vi "Process Libraries.vi"(8 "error in (no error)":errorcluster {"code" format="Error %.0f"}, 10 "Libraries":refnum<class "Library Documentation.lvclass">[](array[class]), 11 "VIDoc Printer In":refnum<class "VIDoc Printer.lvclass">) -> (0 "error out":errorcluster {"code" format="Error %.0f"}, 3 "VIDoc Printer Out":refnum<class "VIDoc Printer.lvclass">)   [LabVIEW 2023, in "VIDoc Printer.lvlib" / "VIDoc Printer.lvclass"]
uses:
  VIDoc Printer.lvclass
  VIDoc Printer.lvclass/VIDoc Printer.ctl
  Parsing/Library Documentation/Library Documentation.lvclass
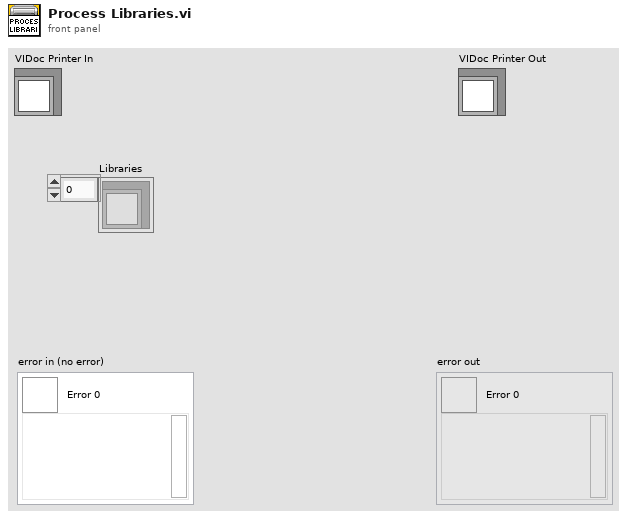
[diagram p1: front panel]
types:
  T1 = typedef "VIDoc Printer.lvlib/VIDoc Printer.lvclass/Process Library Enum.ctl" = enum16{"Header", "Memory", "By Folder", "By Tree", "By List", "Description", "Properties", "Child Libraries", "Friends", "Methods", "Controls"}
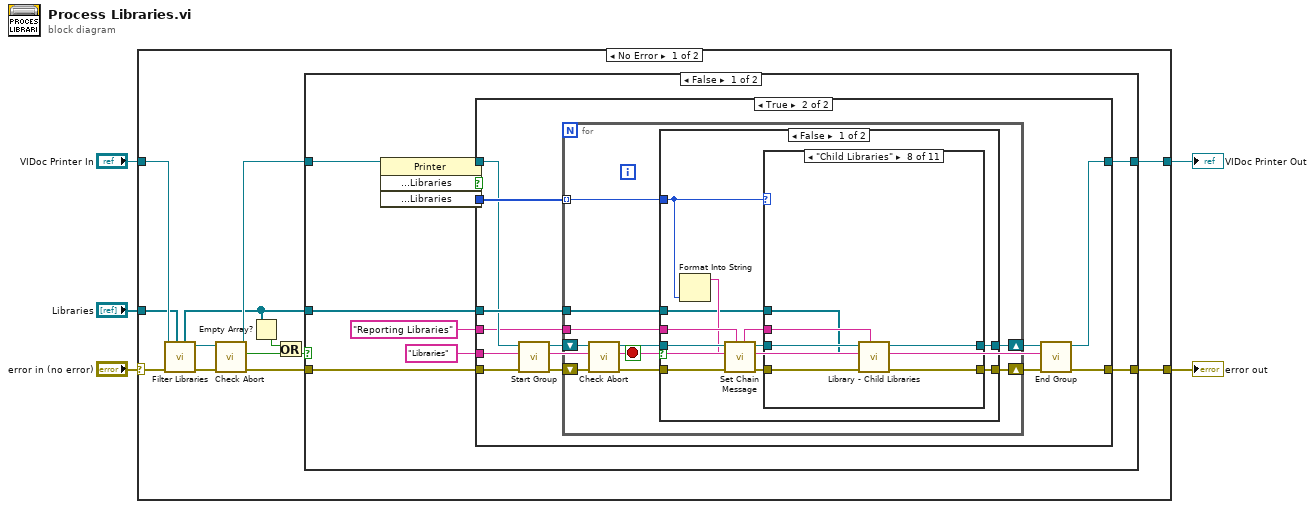
[diagram p0: block diagram]
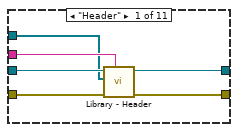
[diagram p3: hidden frame]
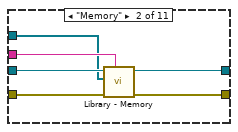
[diagram p4: hidden frame]
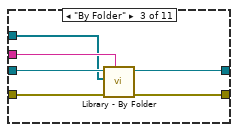
[diagram p5: hidden frame]
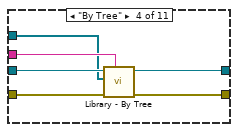
[diagram p6: hidden frame]
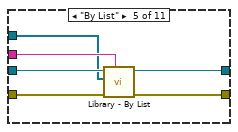
[diagram p7: hidden frame]
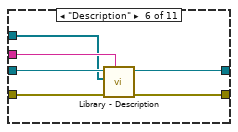
[diagram p8: hidden frame]
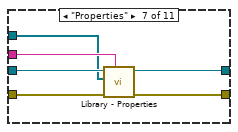
[diagram p9: hidden frame]
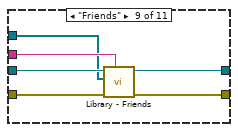
[diagram p10: hidden frame]
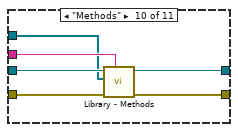
[diagram p11: hidden frame]
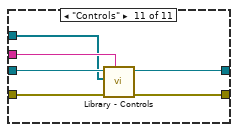
[diagram p12: hidden frame]
diagram:
  n1 = case shown="No Error" "error in (no error)" {
    selector: "error in (no error)" -> [w18 w135]
    tunnel: [w14 w135] -> w2
    tunnel: [w13 w134] -> w1
    tunnel: "VIDoc Printer In" -> [w8 w134]
    tunnel: "Libraries" -> [w6 _]
    frame No Error {
      n2 = call "Filter Libraries.vi"("Libraries"=w6, "error in (no error)"=w18, "VIDoc Printer In"=w8) -> ("error out"=w10:errorcluster, "VIDoc Printer Out"=w9:refnum<class "VIDoc Printer.lvclass">, "Filtered Libraries"=w7:refnum<class "Library Documentation.lvclass">[])  [unwired: 6 in]
      n3 = call "Check Abort.vi"("error in (no error)"=w10, "VIDoc Printer In"=w9) -> ("error out"=w17:errorcluster, "Abort?"=w15:bool, "VIDoc Printer Out"=w16:refnum<class "VIDoc Printer.lvclass">)  [unwired: 7 in]
      n4 = Empty Array?(array=w7) -> (empty?=w11:bool)
      n5 = Or(x=w11, y=w15) -> (x .or. y?=w12:bool)
      n6 = case shown="False" w12 {
        tunnel: w7 -> [w28 _]
        tunnel: w17 -> [w25 w133]
        tunnel: w16 -> [w26 w132]
        tunnel: [w23 w133] -> w14
        tunnel: [w24 w132] -> w13
        frame False {
          n7 = property class="Printer"(reference=w26) -> (reference out=w27:refnum<class "VIDoc Printer.lvclass">, "Properties:Settings:Enabled Sections:Libraries"=w20:bool, "Properties:Process Lists:Libraries"=w19:T1[])  [unwired: 1 in, 1 out]
          n8 = case shown="True" w20 {
            tunnel: w25 -> [w30 w40]
            tunnel: "Reporting Libraries" ("Section") -> [_ w32]
            tunnel: [w30 w33] -> w23
            tunnel: w28 -> [_ w42]
            tunnel: w27 -> [w29 w37]
            tunnel: [w29 w34] -> w24
            tunnel: w19 -> [_ w41]
            tunnel: "Libraries" ("Section") -> [_ w31]
            frame False {
            }
            frame True {
              n9 = call-dynamic "Start Group.vi"("error in (no error)"=w40, "Group"=w31, "VIDoc Printer In"=w37) -> ("error out"=w39:errorcluster, "VIDoc Printer Out"=w38:refnum<class "VIDoc Printer.lvclass">)  [unwired: 7 in]
              n10 = for {
                shift-right: [w50] -> w35
                shift-left: w39 -> [w52]
                tunnel: w32 -> [w46]
                tunnel: w42 -> [w45]
                shift-right: [w48] -> w36
                shift-left: w38 -> [w51]
                tunnel: w41 -> [w44] mode=indexing
                stop <- w43 stop-if-true
                n11 = call "Check Abort.vi"("error in (no error)"=w52, "VIDoc Printer In"=w51) -> ("error out"=w49:errorcluster, "Abort?"=w43:bool, "VIDoc Printer Out"=w47:refnum<class "VIDoc Printer.lvclass">)  [unwired: 7 in]
                n12 = case shown="False" w43 {
                  tunnel: [w63 w131] -> w50
                  tunnel: w49 -> [w60 w131]
                  tunnel: [w62 w130] -> w48
                  tunnel: w47 -> [w58 w130]
                  tunnel: w46 -> [w57 _]
                  tunnel: w45 -> [w54 _]
                  tunnel: w44 -> [w56 _]
                  frame False {
                    n13 = Format Into String(w56) -> (resulting string=w55:string)  [unwired: 3 in, 1 out]
                    n14 = call "Set Chain Message.vi"("Msg Chain"=w57, "error in (no error)"=w60, "New"=w55, "VIDoc Printer In"=w58) -> ("error out"=w61:errorcluster, "VIDoc Printer Out"=w59:refnum<class "VIDoc Printer.lvclass">, "Msg Chain out"=w53:string)  [unwired: 5 in]
                    n15 = case shown="\"Child Libraries\"" w56 {
                      tunnel: w61 -> [w68 w74 w80 w86 w92 w98 w104 w111 w116 w122 w128]
                      tunnel: [w66 w72 w78 w84 w90 w96 w102 w110 w114 w120 w126] -> w63
                      tunnel: w59 -> [w69 w75 w81 w87 w93 w99 w105 w109 w117 w123 w129]
                      tunnel: [w67 w73 w79 w85 w91 w97 w103 w108 w115 w121 w127] -> w62
                      tunnel: w54 -> [w64 w70 w76 w82 w88 w94 w100 w106 w112 w118 w124]
                      tunnel: w53 -> [w65 w71 w77 w83 w89 w95 w101 w107 w113 w119 w125]
                      frame "Header" {
                        n16 = call-dynamic "Library - Header.vi"("Msg Chain"=w65, "error in (no error)"=w68, "Libraries"=w64, "VIDoc Printer In"=w69) -> ("error out"=w66:errorcluster, "VIDoc Printer Out"=w67:refnum<class "VIDoc Printer.lvclass">)  [unwired: 6 in]
                      }
                      frame "Memory" {
                        n17 = call-dynamic "Library - Memory.vi"("Msg Chain"=w71, "error in (no error)"=w74, "Libraries"=w70, "VIDoc Printer In"=w75) -> ("error out"=w72:errorcluster, "VIDoc Printer Out"=w73:refnum<class "VIDoc Printer.lvclass">)  [unwired: 6 in]
                      }
                      frame "By Folder" {
                        n18 = call-dynamic "Library - By Folder.vi"("Msg Chain"=w77, "error in (no error)"=w80, "Libraries"=w76, "VIDoc Printer In"=w81) -> ("error out"=w78:errorcluster, "VIDoc Printer Out"=w79:refnum<class "VIDoc Printer.lvclass">)  [unwired: 6 in]
                      }
                      frame "By Tree" {
                        n19 = call-dynamic "Library - By Tree.vi"("Msg Chain"=w83, "error in (no error)"=w86, "Libraries"=w82, "VIDoc Printer In"=w87) -> ("error out"=w84:errorcluster, "VIDoc Printer Out"=w85:refnum<class "VIDoc Printer.lvclass">)  [unwired: 6 in]
                      }
                      frame "By List" {
                        n20 = call-dynamic "Library - By List.vi"("Msg Chain"=w89, "error in (no error)"=w92, "Libraries"=w88, "VIDoc Printer In"=w93) -> ("error out"=w90:errorcluster, "VIDoc Printer Out"=w91:refnum<class "VIDoc Printer.lvclass">)  [unwired: 6 in]
                      }
                      frame "Description" {
                        n21 = call-dynamic "Library - Description.vi"("Msg Chain"=w95, "error in (no error)"=w98, "Libraries"=w94, "VIDoc Printer In"=w99) -> ("error out"=w96:errorcluster, "VIDoc Printer Out"=w97:refnum<class "VIDoc Printer.lvclass">)  [unwired: 6 in]
                      }
                      frame "Properties" {
                        n22 = call-dynamic "Library - Properties.vi"("Msg Chain"=w101, "error in (no error)"=w104, "Libraries"=w100, "VIDoc Printer In"=w105) -> ("error out"=w102:errorcluster, "VIDoc Printer Out"=w103:refnum<class "VIDoc Printer.lvclass">)  [unwired: 6 in]
                      }
                      frame "Child Libraries" {
                        n23 = call-dynamic "Library - Child Libraries.vi"("Msg Chain"=w107, "error in (no error)"=w111, "Libraries"=w106, "VIDoc Printer In"=w109) -> ("error out"=w110:errorcluster, "VIDoc Printer Out"=w108:refnum<class "VIDoc Printer.lvclass">)  [unwired: 6 in]
                      }
                      frame "Friends" {
                        n24 = call-dynamic "Library - Friends.vi"("Msg Chain"=w113, "error in (no error)"=w116, "Libraries"=w112, "VIDoc Printer In"=w117) -> ("error out"=w114:errorcluster, "VIDoc Printer Out"=w115:refnum<class "VIDoc Printer.lvclass">)  [unwired: 6 in]
                      }
                      frame "Methods" {
                        n25 = call-dynamic "Library - Methods.vi"("Msg Chain"=w119, "error in (no error)"=w122, "Libraries"=w118, "VIDoc Printer In"=w123) -> ("error out"=w120:errorcluster, "VIDoc Printer Out"=w121:refnum<class "VIDoc Printer.lvclass">)  [unwired: 6 in]
                      }
                      frame "Controls" {
                        n26 = call-dynamic "Library - Controls.vi"("Msg Chain"=w125, "error in (no error)"=w128, "Libraries"=w124, "VIDoc Printer In"=w129) -> ("error out"=w126:errorcluster, "VIDoc Printer Out"=w127:refnum<class "VIDoc Printer.lvclass">)  [unwired: 6 in]
                      }
                    }
                  }
                  frame True {
                  }
                }
              }
              n27 = call-dynamic "End Group.vi"("error in (no error)"=w35, "Group"=w31, "VIDoc Printer In"=w36) -> ("error out"=w33:errorcluster, "VIDoc Printer Out"=w34:refnum<class "VIDoc Printer.lvclass">)  [unwired: 7 in]
            }
          }
        }
        frame True {
        }
      }
    }
    frame Error {
    }
  }
  "error out" <- w2
  "VIDoc Printer Out" <- w1
